vi "Set Data Out.vi"   [LabVIEW 2019, in "HD44780.lvlib"]
uses:
  HD44780.lvlib
  <vilib>/rvi/eio/common/nirviEmuTemplateMethod_errors.vi
  <vilib>/eio/EIOMethodNode/EIOMethodNode.xnode
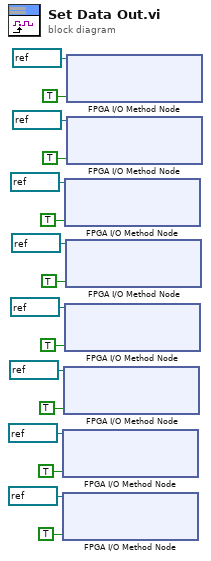
[diagram p0: block diagram]
diagram:
  n1 = xnode "FPGA I/O Method Node"("FPGA I/O In"=refnum<k21> "DB6", "Enable"=TRUE) -> ()  [unwired: 1 out]
  n2 = xnode "FPGA I/O Method Node"("FPGA I/O In"=refnum<k21> "DB7", "Enable"=TRUE) -> ()  [unwired: 1 out]
  n3 = xnode "FPGA I/O Method Node"("FPGA I/O In"=refnum<k21> "DB5", "Enable"=TRUE) -> ()  [unwired: 1 out]
  n4 = xnode "FPGA I/O Method Node"("FPGA I/O In"=refnum<k21> "DB2", "Enable"=TRUE) -> ()  [unwired: 1 out]
  n5 = xnode "FPGA I/O Method Node"("FPGA I/O In"=refnum<k21> "DB4", "Enable"=TRUE) -> ()  [unwired: 1 out]
  n6 = xnode "FPGA I/O Method Node"("FPGA I/O In"=refnum<k21> "DB3", "Enable"=TRUE) -> ()  [unwired: 1 out]
  n7 = xnode "FPGA I/O Method Node"("FPGA I/O In"=refnum<k21> "DB0", "Enable"=TRUE) -> ()  [unwired: 1 out]
  n8 = xnode "FPGA I/O Method Node"("FPGA I/O In"=refnum<k21> "DB1", "Enable"=TRUE) -> ()  [unwired: 1 out]
